vi "calculate rgb with encoded ascii.vi"(8 "original r":u8, 9 "original g":u8, 10 "original b":u8, 11 "ch as u8":u8) -> (0 "new r":u8, 1 "new g":u8, 2 "new b":u8)   [LabVIEW 2020]
doc: "Takes the orignal b, g, and r components as a u8 and inserts <b>ch as u8</b> across the LSBs of each component.\n\nFor example, if the <b>ch as u8</b> is 97 (for 'a'), then its 7 bits are 1100001b (MSB....LSBb). This is split into 11b, 00b, and 001b which will be inserted into the red, green, and blue components' LSBs.\n\nIf the original blue value was 125d (01111101b), then the original lower bits 101b will be converted to 001b. The new blue value is then 01111001b (121d).\n\nIf the original green value was 254d (11111110b), then the original lower bits 10b will be converted to 00b. The new green value is then 11111100b (252d).\n\nIf the original red value was 7d (00000111b), then the original lower bits 11b will be converted to 11b (technically, no change needed!). The new red value is then 00000111b (7d)."
panel:
  out "new r array":bool[](array[boolean])
  out "new g array":bool[](array[boolean])
  out "new b array":bool[](array[boolean])
  out "original r array":bool[](array[boolean])
  out "original g array":bool[](array[boolean])
  out "original b array":bool[](array[boolean])
  out "red bits":bool[](array[boolean])
  out "green bits":bool[](array[boolean])
  out "blue bits":bool[](array[boolean])
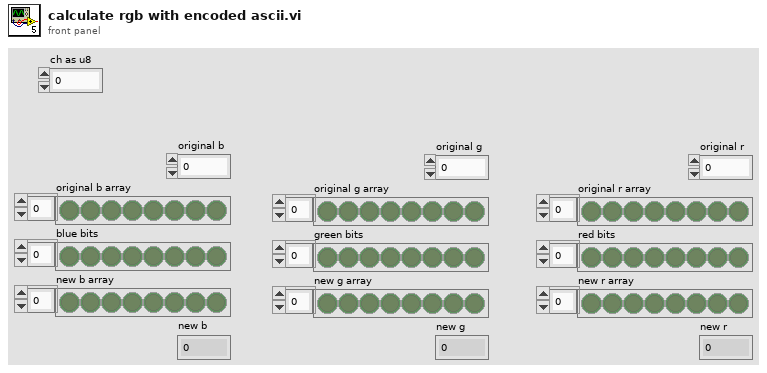
[diagram p1: front panel]
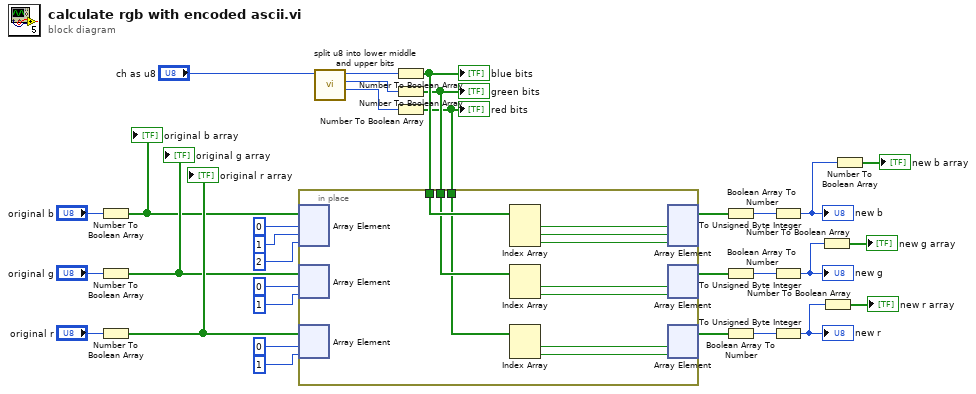
[diagram p0: block diagram]
diagram:
  n1 = Number To Boolean Array(number="original b") -> (Boolean array=w24:bool[])
  "original b array" <- w24
  n2 = Number To Boolean Array(number="original g") -> (Boolean array=w25:bool[])
  "original g array" <- w25
  n3 = Number To Boolean Array(number="original r") -> (Boolean array=w26:bool[])
  "original r array" <- w26
  n4 = call "split u8 into lower middle and upper bits.vi"("Numeric"="ch as u8") -> ("upper 2 bits as number for red"=w29:u8, "middle 2 bits as number for green"=w28:u8, "lower 3 bits as number for blue"=w27:u8)  [unwired: 8 in]
  n5 = Number To Boolean Array(number=w27) -> (Boolean array=w19:bool[])
  "blue bits" <- w19
  n6 = Number To Boolean Array(number=w28) -> (Boolean array=w18:bool[])
  "green bits" <- w18
  n7 = Number To Boolean Array(number=w29) -> (Boolean array=w17:bool[])
  "red bits" <- w17
  n8 = in-place {
    in-place-border: w19 -> [w42]
    in-place-border: w18 -> [w41]
    in-place-border: w17 -> [w40]
    n9 = in-place-array #1(w24, 0, 1, 2) -> ()  [unwired: 3 out]
    n10 = in-place-array #2(w25, 0, 1) -> ()  [unwired: 2 out]
    n11 = in-place-array #3(w26, 0, 1) -> ()  [unwired: 2 out]
    n12 = Index Array(array=w42) -> (element #1=w39:bool, element #2=w38:bool, element #3=w37:bool)  [unwired: 3 in]
    n13 = Index Array(array=w41) -> (element #1=w36:bool, element #2=w35:bool)  [unwired: 2 in]
    n14 = Index Array(array=w40) -> (element #1=w34:bool, element #2=w33:bool)  [unwired: 2 in]
    n15 = in-place-array #1(w39, w38, w37) -> (w20:bool[])  [unwired: 3 out]
    n16 = in-place-array #2(w36, w35) -> (w15:bool[])  [unwired: 2 out]
    n17 = in-place-array #3(w34, w33) -> (w16:bool[])  [unwired: 2 out]
  }
  n18 = Boolean Array To Number(Boolean array=w20) -> (number=w23:u32)
  n19 = Boolean Array To Number(Boolean array=w15) -> (number=w22:u32)
  n20 = Boolean Array To Number(Boolean array=w16) -> (number=w21:u32)
  n21 = To Unsigned Byte Integer(number=w23) -> (unsigned 8bit integer=w7:u8)
  "new b" <- w7
  n22 = To Unsigned Byte Integer(number=w22) -> (unsigned 8bit integer=w5:u8)
  "new g" <- w5
  n23 = To Unsigned Byte Integer(number=w21) -> (unsigned 8bit integer=w3:u8)
  "new r" <- w3
  n24 = Number To Boolean Array(number=w5) -> (Boolean array=→"new g array":bool[])
  n25 = Number To Boolean Array(number=w3) -> (Boolean array=→"new r array":bool[])
  n26 = Number To Boolean Array(number=w7) -> (Boolean array=→"new b array":bool[])
